vi "Logger.ReadVariable.vi"(8 "error in (no error)":errorcluster, 9 "Data":variant, 10 "Address":string, 11 "Logger":refnum<class "Logger.lvclass">) -> (0 "error out":errorcluster, 3 "Logger out":refnum<class "Logger.lvclass">)   [LabVIEW 2016, in "Logger.lvclass"]
doc: "---------------------------------------------------------------\nJKI State Machine Objects™\nhttp://jki.net/state-machine-objects/\nCopyright (C) 2005-2015, JKI <info@jki.net>\nALL RIGHTS RESERVEDJKI State Machine Objects (SMO) 1.0.0.4\nJKI - JKI\nCopyright (c) 2015, JKI"
uses:
  Logger.lvclass
  Typedefs/PublicEvents--Logger.Read Variable.ctl
  Logger.lvclass/Logger.ctl
panel:
  # "For instructions on how to use the JKI State Machine Objects, examples and video tutorials, visit:\nhttp://jki.net/state-machine-objects/\n\nJKI State Machine Objects™\nhttp://jki.net/state-machine-objects/\nCopyright (C) 2005-2015, JKI <info@jki.net>\nALL RIGHTS RESERVED"
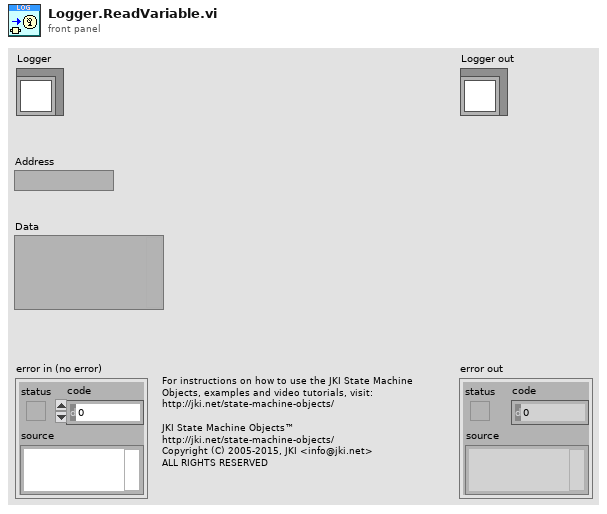
[diagram p1: front panel]
types:
  T1 = typedef "Logger.lvclass/PublicEvents--Logger.Read Variable.ctl" = cluster{"Address":string, "Data":variant}
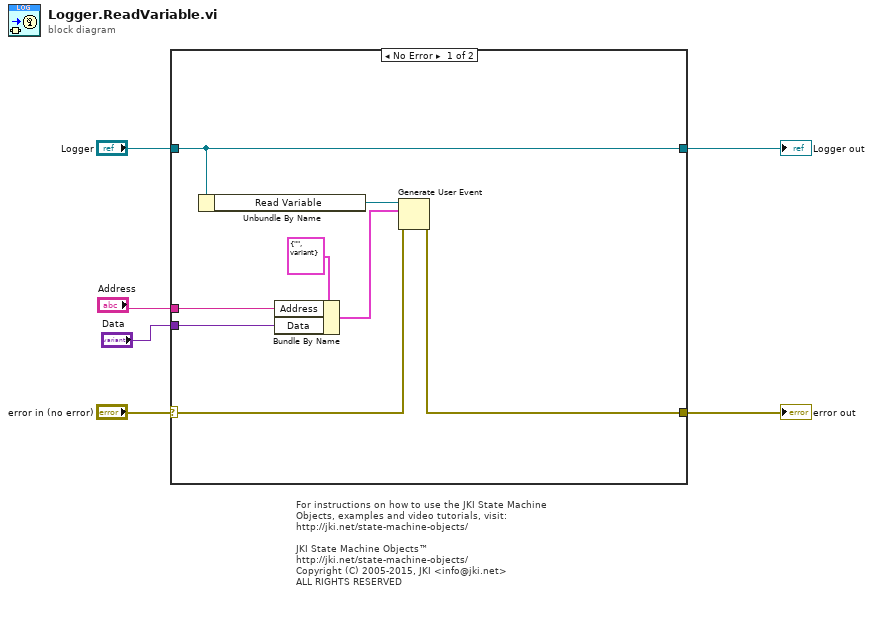
[diagram p0: block diagram]
diagram:
  # "For instructions on how to use the JKI State Machine Objects, examples and video tutorials, visit:\nhttp://jki.net/state-machine-objects/\n\nJKI State Machine Objects™\nhttp://jki.net/state-machine-objects/\nCopyright (C) 2005-2015, JKI <info@jki.net>\nALL RIGHTS RESERVED"
  n1 = case shown="No Error" "error in (no error)" {
    selector: "error in (no error)" -> [w14 w16]
    tunnel: [w12 w16] -> w5
    tunnel: [w11 w15] -> w6
    tunnel: "Logger" -> [w11 w15]
    tunnel: "Address" -> [w9 _]
    tunnel: "Data" -> [w8 _]
    frame No Error {
      n2 = Unbundle By Name(w11) -> ("Read Variable"=w13:refnum<user-event>)
      n3 = Bundle By Name(cluster=T1 {"Address"="", "Data"=variant} ("Write Variable"), "Address"=w9, "Data"=w8) -> (w7:T1)
      n4 = Generate User Event(user event=w13, event data cluster=w7, error in=w14) -> (error out=w12:errorcluster)  [unwired: 1 in, 1 out]
    }
    frame Error {
    }
  }
  "error out" <- w5
  "Logger out" <- w6
